vi "Stop Nested Models.vi"(8 "error in (no error)":errorcluster, 10 "Stop Msg":refnum<class "Stop Msg.lvclass">, 11 "IModel in":refnum<class "IModel.lvclass">) -> (0 "error out":errorcluster, 2 "Tracked Actors Running":i32, 3 "IModel out":refnum<class "IModel.lvclass">)   [LabVIEW 2018, in "MVA Framework.lvlib" / "IModel.lvlib" / "IModel.lvclass"]
doc: "停止嵌套模型"
uses:
  IModel.lvclass
  <vilib>/ActorFramework/Message Enqueuer/Message Enqueuer.lvclass
  <vilib>/ActorFramework/Stop Msg/Stop Msg.lvclass
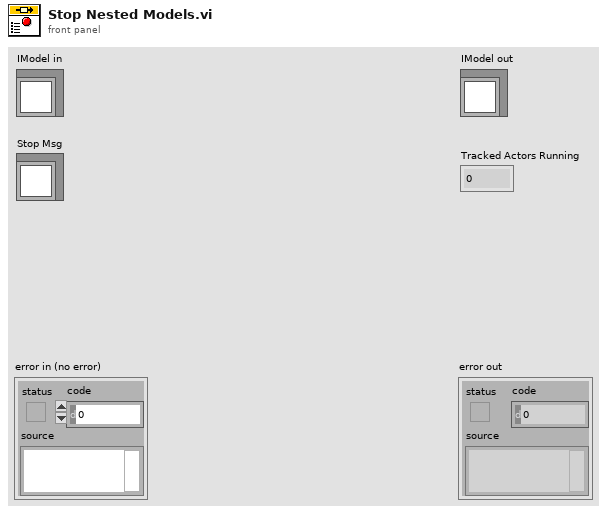
[diagram p1: front panel]
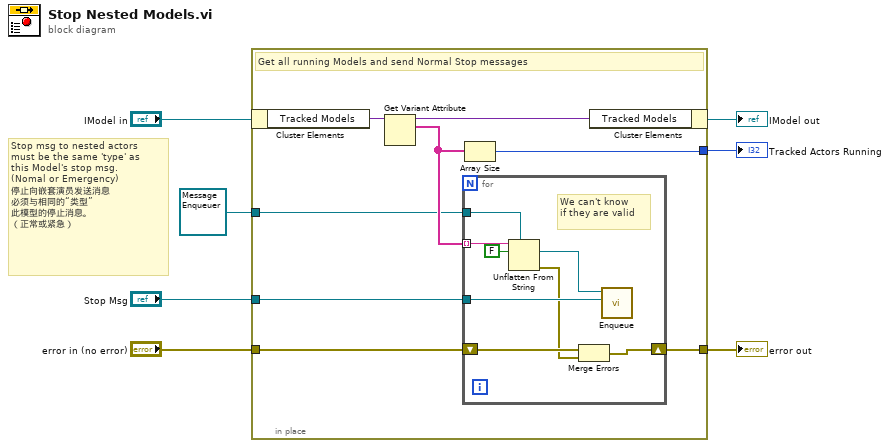
[diagram p0: block diagram]
diagram:
  # "Stop msg to nested actors\nmust be the same 'type' as\nthis Model's stop msg.\n(Nomal or Emergency)\n停止向嵌套演员发送消息\n必须与相同的“类型”\n此模型的停止消息。\n（正常或紧急）"
  n1 = in-place {
    in-place-border: refnum<class "Message Enqueuer.lvclass"> refnum ("Nested Model Enqueuer") -> [w8]
    in-place-border: "error in (no error)" -> [w13]
    in-place-border: [w12] -> w3
    in-place-border: [w10] -> w2
    in-place-border: "Stop Msg" -> [w9]
    # "Get all running Models and send Normal Stop messages"
    n2 = in-place-cluster #1("IModel in") -> ("Tracked Models"=w15:variant)
    n3 = Get Variant Attribute(Variant=w15) -> (duplicate Variant=w14:variant, names=w11:string[])  [unwired: 3 in, 2 out]
    n4 = for {
      tunnel: w8 -> [w22]
      tunnel: w11 -> [w21] mode=indexing
      shift-right: [w19] -> w12
      shift-left: w13 -> [w18]
      tunnel: w9 -> [w23]
      # "We can't know\nif they are valid"
      n5 = Unflatten From String(type=w22, binary string=w21, data includes array or string size? (T)=FALSE) -> (value=w16:refnum<class "Message Enqueuer.lvclass">, error out=w17:errorcluster)  [unwired: 2 in, 1 out]
      n6 = Merge Errors(w18, w17) -> (w19:errorcluster)
      n7 = call <vilib>:"Enqueue.vi"("Message"=w23, "Message Enqueuer in"=w16) -> ()  [unwired: 8 in, 2 out]
    }
    n8 = Array Size(array=w11) -> (size(s)=w10:i32)
    n9 = in-place-cluster #1("Tracked Models"=w14) -> (→"IModel out":refnum<class "IModel.lvclass">)
  }
  "error out" <- w3
  "Tracked Actors Running" <- w2
